vi "FilterLowPassX(SubVI_Exo2).vi"(8 "error in (no error)":errorcluster, 11 "X-Axis":dbl) -> (0 "error out":errorcluster, 3 "Filtered x":dbl)   [LabVIEW 2019]
uses:
  <vilib>/ptbypt/NI_PtbyPt.lvlib
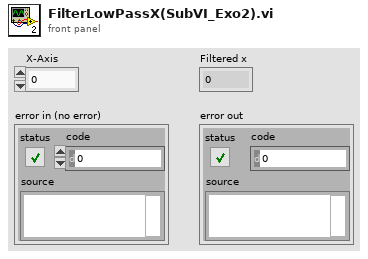
[diagram p1: front panel]
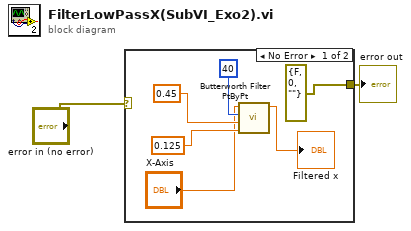
[diagram p0: block diagram]
diagram:
  n1 = case shown="No Error" "error in (no error)" {
    selector: "error in (no error)" -> [_ w9]
    tunnel: [errorcluster {"status"=FALSE, "code"=0, "source"=""} ("error IO") w9] -> w2
    frame No Error {
      n2 = call <vilib>:"Butterworth Filter PtByPt.vi"("low cutoff freq: fl"=0.125, "high cutoff freq: fh"=0.45, "sampling freq: fs"=40, "x"="X-Axis") -> ("Filtered x"=→"Filtered x":dbl)  [unwired: 5 in, 1 out]
    }
    frame Error {
    }
  }
  "error out" <- w2
